vi "Sorted Particle Report Port.vi"(3 "Min Area Size %":dbl, 4 "Particle Count Limit":i32=1, 5 "Pixel Measurements":T2[](array[typedef])=[35, 4, 5, 6, 7] items=["Center of Mass X", "Center of Mass Y", "First Pixel X", "First Pixel Y", "Bounding Rect Left", "Bounding Rect Top", "Bounding Rect Right", "Bounding Rect Bottom", "Max Feret Diameter Start X", "Max Feret Diameter Start Y", "Max Feret Diameter End X", "Max Feret Diameter End Y", "Max Horiz. Segment Length Left", "Max Horiz. Segment Length Right", "Max Horiz. Segment Length Row", "-", "Bounding Rect Width", "Bounding Rect Height", "Bounding Rect Diagonal", "Perimeter", "Convex Hull Perimeter", "Holes' Perimeter", "Max Feret Diameter", "Equivalent Ellipse Major Axis", "Equivalent Ellipse Minor Axis", "Equivalent Ellipse Minor Axis (Feret)", "Equivalent Rect Long Side", "Equivalent Rect Short Side", "Equivalent Rect Diagonal", "Equivalent Rect Short Side (Feret)", "Average Horiz. Segment Length", "Average Vert. Segment Length", "Hydraulic Radius", "Waddel Disk Diameter", "-", "Area", "Holes' Area", "Particle & Holes' Area", "Convex Hull Area", "Image Area", "-", "Number of Holes", "Number of Horiz. Segments", "Number of Vert. Segments", "-", "Orientation", "Max Feret Diameter Orientation", "-", "% Area/Image Area", "% Area/(Particle & Holes' Area)", "Ratio of Equivalent Ellipse Axes", "Ratio of Equivalent Rect Sides", "-", "Elongation Factor", "Compactness Factor", "Heywood Circularity Factor", "Type Factor", "-", "Sum X", "Sum Y", "Sum XX", "Sum XY", "Sum YY", "Sum XXX", "Sum XXY", "Sum XYY", "Sum YYY", "-", "Moment of Inertia XX", "Moment of Inertia XY", "Moment of Inertia YY", "Moment of Inertia XXX", "Moment of Inertia XXY", "Moment of Inertia XYY", "Moment of Inertia YYY", "Norm. Moment of Inertia XX", "Norm. Moment of Inertia XY", "Norm. Moment of Inertia YY", "Norm. Moment of Inertia XXX", "Norm. Moment of Inertia XXY", "Norm. Moment of Inertia XYY", "Norm. Moment of Inertia YYY", "Hu Moment 1", "Hu Moment 2", "Hu Moment 3", "Hu Moment 4", "Hu Moment 5", "Hu Moment 6", "Hu Moment 7"], 6 "Image in":T3) -> (0 "limits":T1, 1 "Sorted Data":dbl[][](array[numeric]), 2 "Particles":i32)   [LabVIEW 2025]
doc: "Returns the requested measurements of a binary image sorted by the first parameter (often size), and limiting the rows in the 2D array by count and by size. Pass infinity to count to avoid a limit. Pass zero to size to avoid a limit."
uses:
  <vilib>/vision/Image Controls.llb/IMAQ Image.ctl
  <vilib>/vision/NI_Vision_Development_Module.lvlib
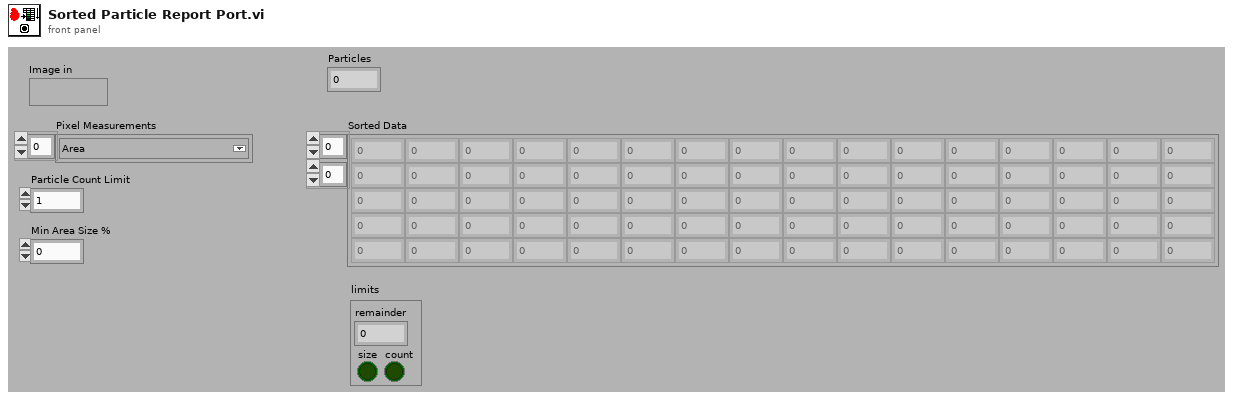
[diagram p1: front panel]
types:
  T1 = cluster{"remainder":i32, "size":bool, "count":bool}
  T2 = typedef "Particle Parameters" = i32
  T3 = typedef "IMAQ Image.ctl" = refnum<image>
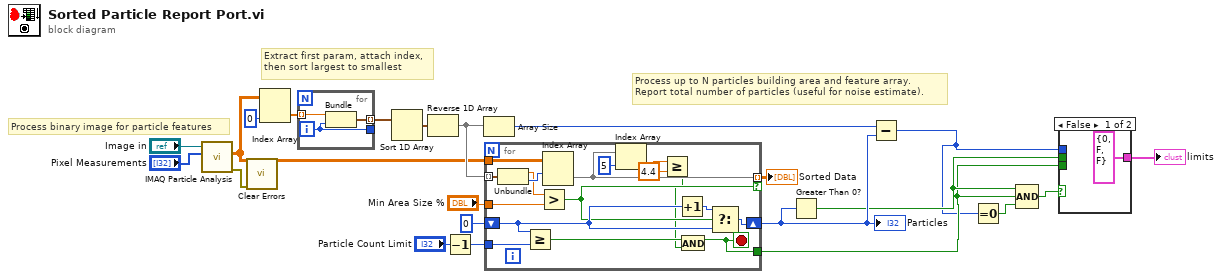
[diagram p0: block diagram]
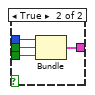
[diagram p2: hidden frame]
diagram:
  # "Process up to N particles building area and feature array.\nReport total number of particles (useful for noise estimate)."
  # "Process binary image for particle features"
  # "Extract first param, attach index,\nthen sort largest to smallest"
  n1 = call "IMAQ Particle Analysis"("Pixel Measurements"="Pixel Measurements", "Image"="Image in") -> ("error out"=w13:errorcluster, "Particle Measurements (Pixels)"=w11:dbl[][])  [unwired: 3 in, 5 out]
  n2 = call <vilib>:"Clear Errors.vi"("error in (no error)"=w13) -> ()  [unwired: 5 in, 2 out]
  n3 = Index Array(array=w11, index (col)=0 ("disabled index (col)")) -> (element=w19:dbl[])  [unwired: 1 in]
  n4 = for {
    tunnel: w19 -> [w25] mode=indexing
    tunnel: [w24] -> w20 mode=indexing
    tunnel: [w23] -> _
    i -> [w23]
    n5 = Bundle("Numeric"=w25, w23) -> (w24:cluster{"Numeric":dbl, i32})  [unwired: 1 out]
  }
  n6 = Sort 1D Array(array=w20) -> (sorted array=w21:cluster{"Numeric":dbl, i32}[])
  n7 = Reverse 1D Array(array=w21) -> (reversed array=w12:cluster{"Numeric":dbl, i32}[])
  n8 = Decrement(x="Particle Count Limit") -> (x-1=w9:i32)
  n9 = Array Size(array=w12) -> (size(s)=w15:i32)
  n10 = for {
    tunnel: w11 -> [w41]
    tunnel: w12 -> [w40] mode=indexing
    tunnel: w9 -> [w39]
    tunnel: "Min Area Size %" -> [w37]
    tunnel: [w31] -> w3
    tunnel: [w30] -> w8 mode=indexing if=w32
    shift-right: [w35] -> w6
    shift-left: 0 -> [w33]
    stop <- w31 stop-if-true
    n11 = Unbundle(w40) -> ("Numeric"=w38:dbl, w42:i32)
    n12 = Greater Or Equal?(x=w33, y=w39) -> (x >= y?=w36:bool)
    n13 = Greater?(x=w38, y=w37) -> (0:w32:bool)
    n14 = Index Array(array=w41, index (row)=w42) -> (element=w30:dbl[])  [unwired: 1 in]
    n15 = Index Array(array=w30, index=5) -> (element=w28:dbl)
    n16 = Greater Or Equal?(x=w28, y=4.4) -> (x >= y?=w26:bool)
    n17 = Increment(x=w33) -> (x+1=w34:i32)
    n18 = And(x=w36, y=w26) -> (x .and. y?=w31:bool)
    n19 = Select(t=w34, s=w32, f=w33) -> (s? t:f=w35:i32)
  }
  "Particles" <- w6
  "Sorted Data" <- w8
  n20 = Greater Than 0?(x=w6) -> (x > 0?=w4:bool)
  n21 = Subtract(x=w15, y=w6) -> (x-y=w2:i32)
  n22 = Equal To 0?(x=w2) -> (x = 0?=w1:bool)
  n23 = Compound Arithmetic op=AND(w4, w3, w1) -> (w5:bool)
  n24 = case shown="False" w5 {
    tunnel: w2 -> [_ w47]
    tunnel: [cluster{i32, bool, bool} {0, FALSE, FALSE} w46] -> w14
    tunnel: w3 -> [_ w45]
    tunnel: w4 -> [_ w44]
    frame False {
    }
    frame True {
      n25 = Bundle(w47, w44, w45) -> (w46:cluster{i32, bool, bool})  [unwired: 1 in]
    }
  }
  "limits" <- w14
